vi "Unflatten.vi"(8 "error in":errorcluster, 10 "Buffer":u8[](array[numeric]) format="%.0x") -> (0 "error out":errorcluster, 2 "Data":T1)   [LabVIEW 2020, in "TcpClientInfo.lvlib"]
uses:
  TcpClientInfo.lvlib
  Data.ctl
  lv-protoc/LV-Proto/Wire Decode Varint I32.vi
  lv-protoc/LV-Proto/Extract Varint Bytes.vi
  lv-protoc/LV-Proto/LV-Proto.lvlib
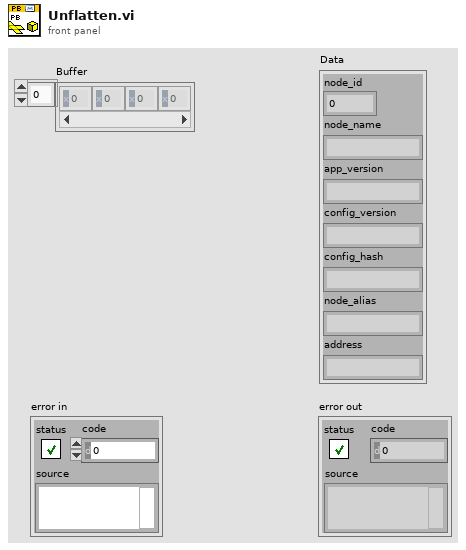
[diagram p1: front panel]
types:
  T1 = typedef "TcpClientInfo.lvlib/Data.ctl" = cluster{"node_id":u32, "node_name":string, "app_version":string, "config_version":string, "config_hash":string, "node_alias":string, "address":string}
  T2 = typedef "LV-Proto.lvlib/Wire Type.ctl" = enum8{"VARINT", "I64", "LEN", "SGROUP (Deprecated)", "EGROUP (Deprecated)", "I32"}
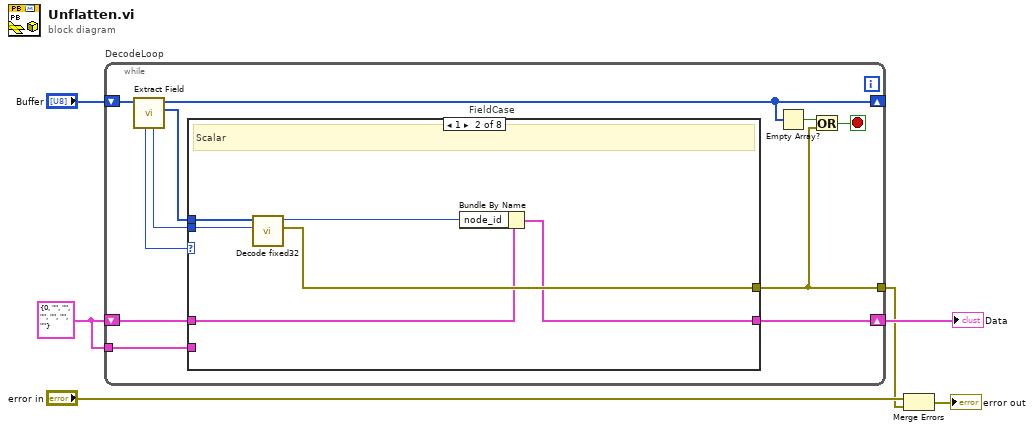
[diagram p0: block diagram]
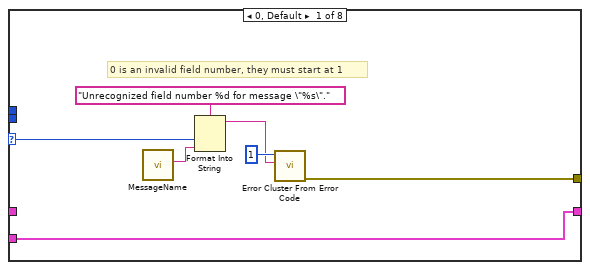
[diagram p2: hidden frame]
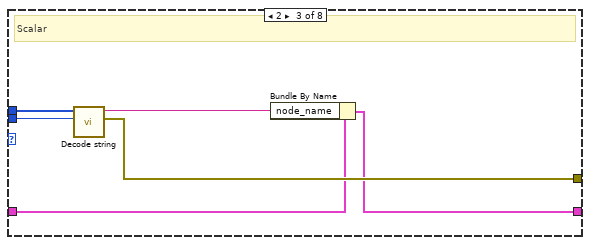
[diagram p3: hidden frame]
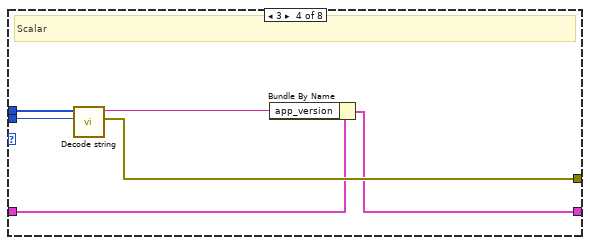
[diagram p4: hidden frame]
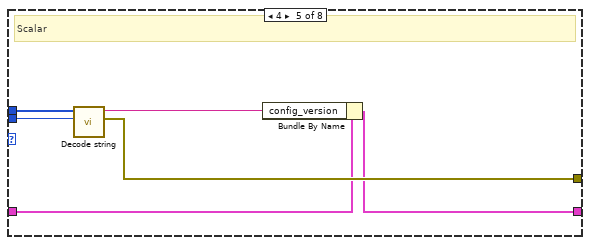
[diagram p5: hidden frame]
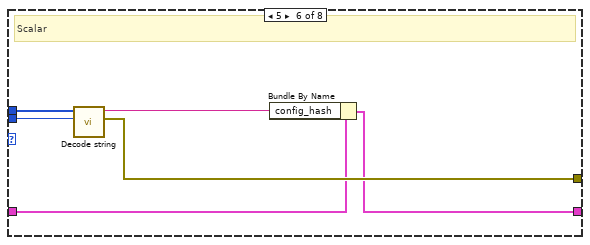
[diagram p6: hidden frame]
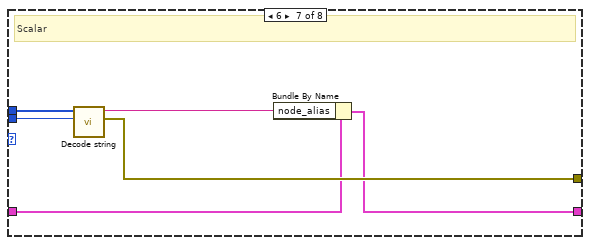
[diagram p7: hidden frame]
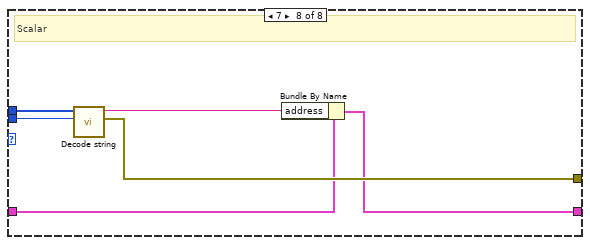
[diagram p8: hidden frame]
diagram:
  w4 = T1 {"node_id"=0, "node_name"="", "app_version"="", "config_version"="", "config_hash"="", "node_alias"="", "address"=""} ("Data")
  n1 = while "DecodeLoop" {
    shift-right: [w16] -> _
    shift-left: "Buffer" -> [w17]
    shift-right: [w9] -> w5
    shift-left: w4 -> [w15]
    tunnel: [w8] -> w2
    tunnel: w4 -> [w7]
    stop <- w11 stop-if-true
    n2 = call "Extract Field.vi"("Buffer in"=w17) -> ("Field Data"=w10:u8[], "Buffer"=w16:u8[], "Wire Type"=w13:T2, "Field Number"=w14:i32)  [unwired: 7 in]
    n3 = case "FieldCase" shown="1" w14 {
      selector: w14 -> [w23 _ _ _ _ _ _ _]
      tunnel: w15 -> [_ w26 w32 w38 w44 w50 w56 w62]
      tunnel: w13 -> [_ w28 w34 w40 w46 w52 w58 w64]
      tunnel: w10 -> [_ w29 w35 w41 w47 w53 w59 w65]
      tunnel: [w19 w25 w31 w37 w43 w49 w55 w61] -> w9
      tunnel: [w20 w30 w36 w42 w48 w54 w60 w66] -> w8
      tunnel: w7 -> [w19 _ _ _ _ _ _ _]
      frame 0, Default {
        # "0 is an invalid field number, they must start at 1"
        n4 = call "MessageName.vi"() -> ("MessageName"=w18:string)  [unwired: 11 in]
        n5 = Format Into String(format string="Unrecognized field number %d for message \"%s\".", w23, w18) -> (resulting string=w21:string)  [unwired: 2 in, 1 out]
        n6 = call <vilib>:"Error Cluster From Error Code.vi"("error message (\"\")"=w21, "error code (0)"=1) -> ("error out"=w20:errorcluster)  [unwired: 7 in]
      }
      frame 1 {
        # "Scalar"
        n7 = call "Decode fixed32.vi"("Wire Type"=w28, "Data"=w29) -> ("error out"=w30:errorcluster, "fixed32"=w27:u32)  [unwired: 8 in]
        n8 = Bundle By Name(cluster=w26, "node_id"=w27) -> (w25:T1)
      }
      frame 2 {
        # "Scalar"
        n9 = call "Decode string.vi"("Wire Type"=w34, "Data"=w35) -> ("error out"=w36:errorcluster, "string"=w33:string)  [unwired: 8 in]
        n10 = Bundle By Name(cluster=w32, "node_name"=w33) -> (w31:T1)
      }
      frame 3 {
        # "Scalar"
        n11 = call "Decode string.vi"("Wire Type"=w40, "Data"=w41) -> ("error out"=w42:errorcluster, "string"=w39:string)  [unwired: 8 in]
        n12 = Bundle By Name(cluster=w38, "app_version"=w39) -> (w37:T1)
      }
      frame 4 {
        # "Scalar"
        n13 = call "Decode string.vi"("Wire Type"=w46, "Data"=w47) -> ("error out"=w48:errorcluster, "string"=w45:string)  [unwired: 8 in]
        n14 = Bundle By Name(cluster=w44, "config_version"=w45) -> (w43:T1)
      }
      frame 5 {
        # "Scalar"
        n15 = call "Decode string.vi"("Wire Type"=w52, "Data"=w53) -> ("error out"=w54:errorcluster, "string"=w51:string)  [unwired: 8 in]
        n16 = Bundle By Name(cluster=w50, "config_hash"=w51) -> (w49:T1)
      }
      frame 6 {
        # "Scalar"
        n17 = call "Decode string.vi"("Wire Type"=w58, "Data"=w59) -> ("error out"=w60:errorcluster, "string"=w57:string)  [unwired: 8 in]
        n18 = Bundle By Name(cluster=w56, "node_alias"=w57) -> (w55:T1)
      }
      frame 7 {
        # "Scalar"
        n19 = call "Decode string.vi"("Wire Type"=w64, "Data"=w65) -> ("error out"=w66:errorcluster, "string"=w63:string)  [unwired: 8 in]
        n20 = Bundle By Name(cluster=w62, "address"=w63) -> (w61:T1)
      }
    }
    n21 = Empty Array?(array=w16) -> (empty?=w12:bool)
    n22 = Or(x=w12, y=w8) -> (x .or. y?=w11:bool)
  }
  "Data" <- w5
  n23 = Merge Errors("error in", w2) -> (→"error out":errorcluster)
